vi "Read CB object temperature reached.vi"(8 "error in (no error)":errorcluster, 11 "Temperature IR Bricklet in":refnum<class "Temperature IR Bricklet.lvclass">) -> (0 "error out":errorcluster, 2 "CB object temperature reached":refnum<user-event>, 3 "Temperature IR Bricklet out":refnum<class "Temperature IR Bricklet.lvclass">)   [LabVIEW 2011, in "Tinkerforge.lvlib" / "Temperature IR Bricklet.lvclass"]
uses:
  Temperature IR Bricklet.lvclass
  Temperature IR Bricklet.lvclass/Temperature IR Bricklet.ctl
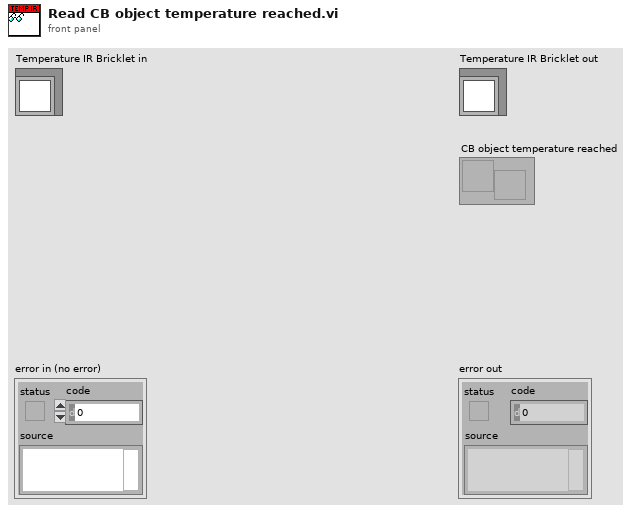
[diagram p1: front panel]
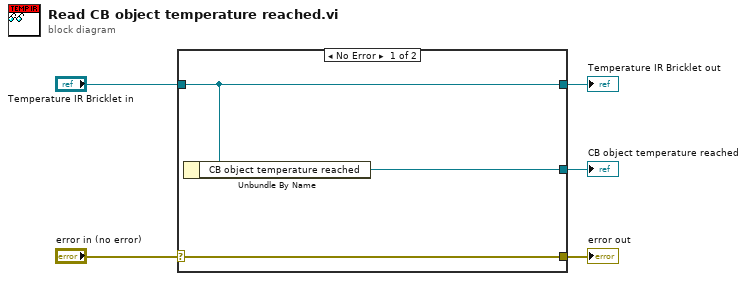
[diagram p0: block diagram]
diagram:
  n1 = case shown="No Error" "error in (no error)" {
    selector: "error in (no error)" -> [w8 w9]
    tunnel: [w8 w9] -> w4
    tunnel: [w7 w10] -> w2
    tunnel: "Temperature IR Bricklet in" -> [w7 w10]
    tunnel: [w6 _] -> w1
    frame No Error {
      n2 = Unbundle By Name(w7) -> ("CB object temperature reached"=w6:refnum<user-event>)
    }
    frame Error {
    }
  }
  "error out" <- w4
  "Temperature IR Bricklet out" <- w2
  "CB object temperature reached" <- w1
